vi "exit_app.vi"(8 "error in (no error)":errorcluster) -> ()   [LabVIEW 2015]
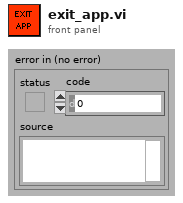
[diagram p1: front panel]
types:
  T1 = enum32{"invalid app kind", "Development System", "Run Time System", "Student Edition", "Embedded LabVIEW", "Evaluation", "Custom"}
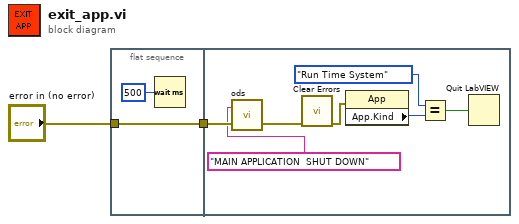
[diagram p0: block diagram]
diagram:
  n1 = flat-sequence {
    tunnel: "error in (no error)" -> [w4]
    tunnel: [w4] -> w1
    tunnel: w1 -> [w8]
    frame #0 {
      n2 = Wait (ms)(milliseconds to wait=u32 500) -> ()  [unwired: 1 out]
    }
    frame #1 {
      n3 = call "ods.vi"("error in (no error)"=w8, "str"="MAIN APPLICATION  SHUT DOWN") -> ("error out"=w6:errorcluster)  [unwired: 1 in]
      n4 = call <vilib>:"Clear Errors.vi"("error in (no error)"=w6) -> ("error out"=w7:errorcluster)  [unwired: 1 in, 5 out]
      n5 = property class="App"(error in=w7) -> ("App.Kind"=w11:T1)  [unwired: 1 in, 2 out]
      n6 = Equal?(x=T1."Run Time System" ("Application:Kind"), y=w11) -> (x = y?=w9:bool)
      n7 = Quit LabVIEW(quit? (T)=w9) -> ()
    }
  }
